vi "Get Test Limits.vi"(10 "Operation Mode":string="Production", 11 "Variant":string="MID") -> (0 "Section6":T1, 1 "Section5":T3, 2 "Section3":T4, 3 "Section2":T5)   [LabVIEW 2025]
uses:
  Controls/Section 2.ctl
  Controls/Limits.ctl
  Controls/Section 3.ctl
  Controls/Section 5.ctl
  Controls/Section 6.ctl
  <vilib>/Utility/file.llb/Read Delimited Spreadsheet (string).vi
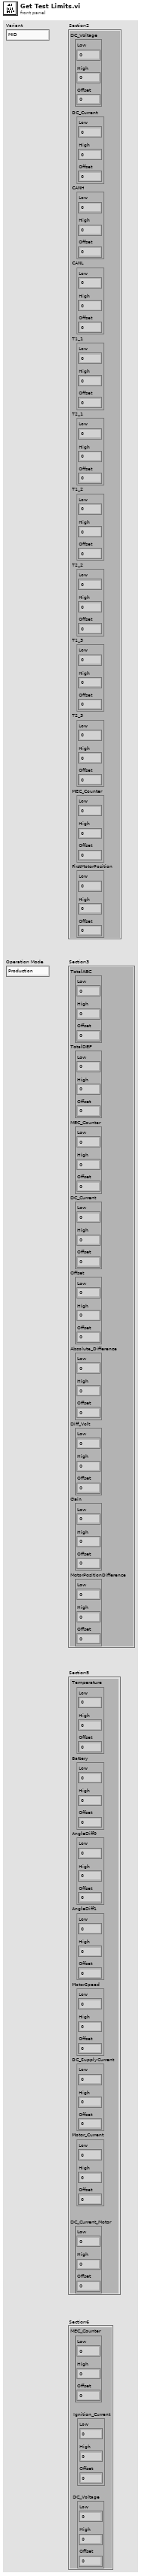
[diagram p1: front panel]
types:
  T1 = typedef "Section 6.ctl" = cluster{"MEC_Counter":T2, "Ignition_Current":T2, "DC_Voltage":T2}
  T2 = typedef "Limits.ctl" = cluster{"Low":dbl, "High":dbl, "Offset":dbl}
  T3 = typedef "Section 5.ctl" = cluster{"Temperature":T2, "Battery":T2, "AngleDiff0":T2, "AngleDiff1":T2, "MotorSpeed":T2, "DC_SupplyCurrent":T2, "Motor_Current":T2, "DC_Current_Motor":T2}
  T4 = typedef "Section 3.ctl" = cluster{"TotalABC":T2, "TotalDEF":T2, "MEC_Counter":T2, "DC_Current":T2, "Offset":T2, "Absolute_Difference":T2, "Diff_Volt":T2, "Gain":T2, "MotorPositionDifference":T2}
  T5 = typedef "Section 2.ctl" = cluster{"DC_Current":T2, "CANH":T2, "CANL":T2, "T1_1":T2, "T2_1":T2, "T1_2":T2, "T2_2":T2, "T1_3":T2, "T2_3":T2, "MEC_Counter":T2, "FirstMotorPosition":T2, "DC_Voltage":T2}
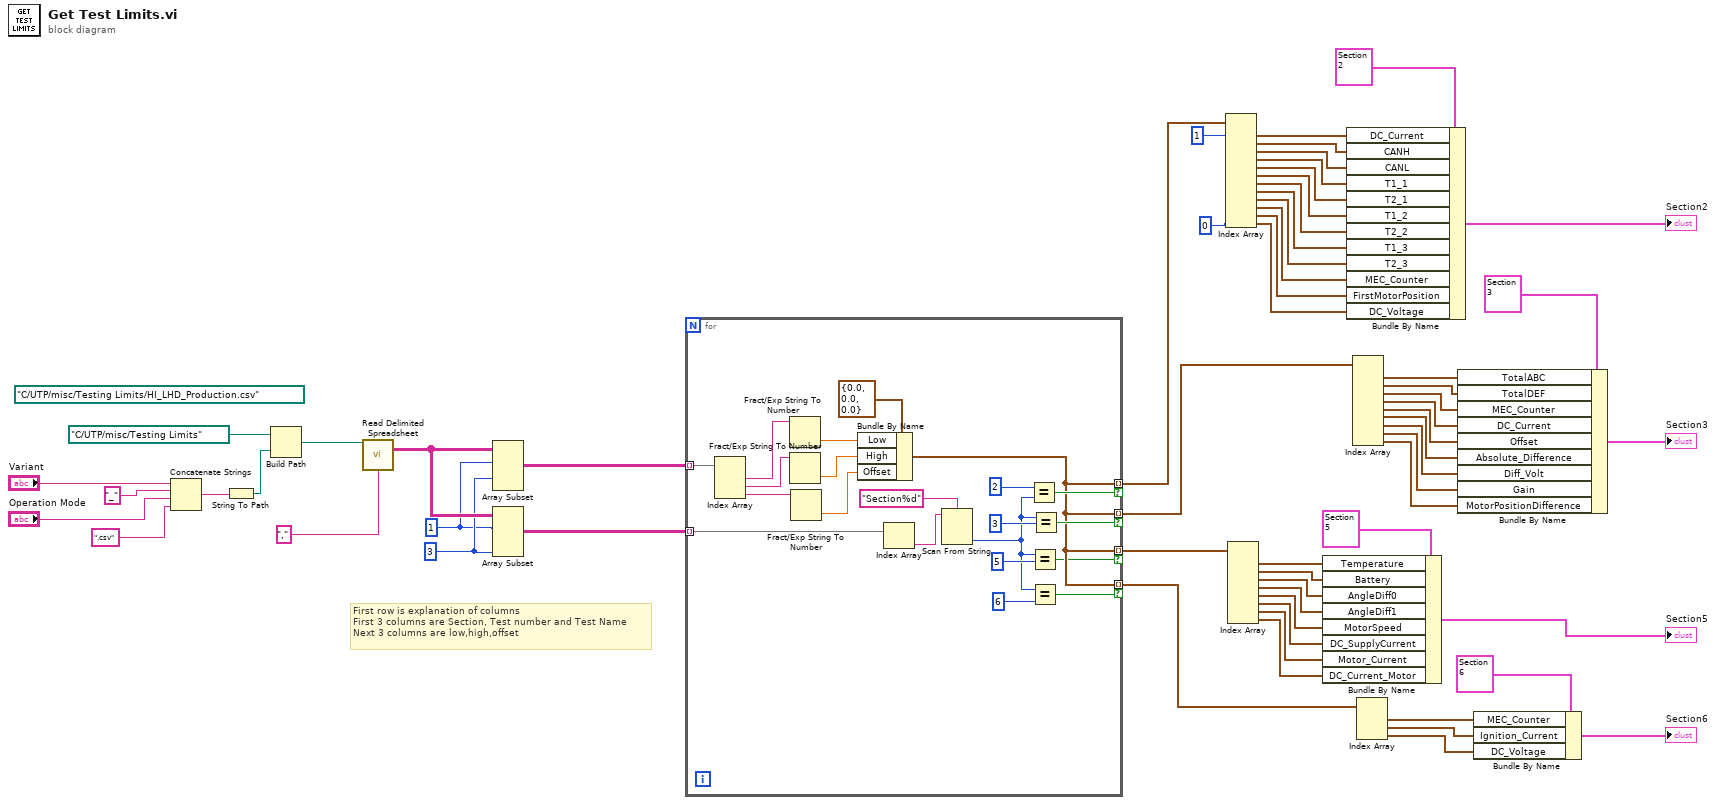
[diagram p0: block diagram]
diagram:
  w57 = 1 ("index")
  w58 = 3 ("index")
  (unwired) path "C:/UTP/misc/Testing Limits/HI_LHD_Production.csv" ("file path (dialog if empty)")
  # "First row is explanation of columns\nFirst 3 columns are Section, Test number and Test Name\nNext 3 columns are low,high,offset"
  n1 = Concatenate Strings("Variant", "_" ("string"), "Operation Mode", ".csv" ("string")) -> (w53:string)
  n2 = String To Path(string=w53) -> (path=w50:path)
  n3 = Build Path(base path=path "C:/UTP/misc/Testing Limits" ("file path (dialog if empty)"), name or relative path=w50) -> (appended path=w49:path)
  n4 = call-poly <vilib>:"Read Delimited Spreadsheet.vi"("file path (dialog if empty)"=w49, "delimiter (\\t)"="," ("delimiter (\\t)")) -> ("all rows"=w59:string[][])  [unwired: 8 in, 5 out]
  n5 = Array Subset(array=w59, index (row)=w57, index (col)=w58) -> (w48:string[][])  [unwired: 2 in]
  n6 = Array Subset(array=w59, index (row)=w57, length (col)=w58) -> (w47:string[][])  [unwired: 2 in]
  n7 = for {
    tunnel: w48 -> [w81] mode=indexing
    tunnel: w47 -> [w77] mode=indexing
    tunnel: [w65] -> w45 mode=indexing if=w69
    tunnel: [w65] -> w32 mode=indexing if=w68
    tunnel: [w65] -> w22 mode=indexing if=w64
    tunnel: [w65] -> w6 mode=indexing if=w61
    n8 = Index Array(array=w81) -> (element #1=w80:string, element #2=w79:string, element #3=w78:string)  [unwired: 3 in]
    n9 = Fract/Exp String To Number(string=w80) -> (number=w72:dbl)  [unwired: 3 in, 1 out]
    n10 = Fract/Exp String To Number(string=w79) -> (number=w71:dbl)  [unwired: 3 in, 1 out]
    n11 = Fract/Exp String To Number(string=w78) -> (number=w70:dbl)  [unwired: 3 in, 1 out]
    n12 = Bundle By Name(cluster=T2 {"Low"=0.0, "High"=0.0, "Offset"=0.0}, "Low"=w72, "High"=w71, "Offset"=w70) -> (w65:T2)
    n13 = Index Array(array=w77) -> (element=w66:string)  [unwired: 1 in]
    n14 = Scan From String(format string="Section%d", input string=w66) -> (output 1=w63:i32)  [unwired: 3 in, 3 out]
    n15 = Equal?(x=2 ("y"), y=w63) -> (x = y?=w69:bool)
    n16 = Equal?(x=w63, y=5) -> (x = y?=w64:bool)
    n17 = Equal?(x=w63, y=6) -> (x = y?=w61:bool)
    n18 = Equal?(x=w63, y=3) -> (x = y?=w68:bool)
  }
  n19 = Index Array(array=w45, index #1=1 ("index"), index #12=0 ("index")) -> (element #1=w44:T2, element #2=w43:T2, element #3=w42:T2, element #4=w41:T2, element #5=w40:T2, element #6=w39:T2, element #7=w38:T2, element #8=w37:T2, element #9=w35:T2, element #10=w36:T2, element #11=w34:T2, element #12=w7:T2)  [unwired: 10 in]
  n20 = Index Array(array=w22) -> (element #1=w20:T2, element #2=w19:T2, element #3=w18:T2, element #4=w17:T2, element #5=w16:T2, element #6=w15:T2, element #7=w14:T2, element #8=w13:T2)  [unwired: 8 in]
  n21 = Bundle By Name(cluster=T3 {"Temperature"={"Low"=0.0, "High"=0.0, "Offset"=0.0}, "Battery"={"Low"=0.0, "High"=0.0, "Offset"=0.0}, "AngleDiff0"={"Low"=0.0, "High"=0.0, "Offset"=0.0}, "AngleDiff1"={"Low"=0.0, "High"=0.0, "Offset"=0.0}, "MotorSpeed"={"Low"=0.0, "High"=0.0, "Offset"=0.0}, "DC_SupplyCurrent"={"Low"=0.0, "High"=0.0, "Offset"=0.0}, "Motor_Current"={"Low"=0.0, "High"=0.0, "Offset"=0.0}, "DC_Current_Motor"={"Low"=0.0, "High"=0.0, "Offset"=0.0}} ("Section5"), "Temperature"=w20, "Battery"=w19, "AngleDiff0"=w18, "AngleDiff1"=w17, "MotorSpeed"=w16, "DC_SupplyCurrent"=w15, "Motor_Current"=w14, "DC_Current_Motor"=w13) -> (→"Section5":T3)
  n22 = Bundle By Name(cluster=T5 {"DC_Current"={"Low"=0.0, "High"=0.0, "Offset"=0.0}, "CANH"={"Low"=0.0, "High"=0.0, "Offset"=0.0}, "CANL"={"Low"=0.0, "High"=0.0, "Offset"=0.0}, "T1_1"={"Low"=0.0, "High"=0.0, "Offset"=0.0}, "T2_1"={"Low"=0.0, "High"=0.0, "Offset"=0.0}, "T1_2"={"Low"=0.0, "High"=0.0, "Offset"=0.0}, "T2_2"={"Low"=0.0, "High"=0.0, "Offset"=0.0}, "T1_3"={"Low"=0.0, "High"=0.0, "Offset"=0.0}, "T2_3"={"Low"=0.0, "High"=0.0, "Offset"=0.0}, "MEC_Counter"={"Low"=0.0, "High"=0.0, "Offset"=0.0}, "FirstMotorPosition"={"Low"=0.0, "High"=0.0, "Offset"=0.0}, "DC_Voltage"={"Low"=0.0, "High"=0.0, "Offset"=0.0}} ("Section2"), "DC_Current"=w44, "CANH"=w43, "CANL"=w42, "T1_1"=w41, "T2_1"=w40, "T1_2"=w39, "T2_2"=w38, "T1_3"=w37, "T2_3"=w35, "MEC_Counter"=w36, "FirstMotorPosition"=w34, "DC_Voltage"=w7) -> (→"Section2":T5)
  n23 = Index Array(array=w32) -> (element #1=w31:T2, element #2=w30:T2, element #3=w29:T2, element #4=w28:T2, element #5=w27:T2, element #6=w26:T2, element #7=w25:T2, element #8=w24:T2, element #9=w23:T2)  [unwired: 9 in]
  n24 = Index Array(array=w6) -> (element #1=w4:T2, element #2=w3:T2, element #3=w2:T2)  [unwired: 3 in]
  n25 = Bundle By Name(cluster=T4 {"TotalABC"={"Low"=0.0, "High"=0.0, "Offset"=0.0}, "TotalDEF"={"Low"=0.0, "High"=0.0, "Offset"=0.0}, "MEC_Counter"={"Low"=0.0, "High"=0.0, "Offset"=0.0}, "DC_Current"={"Low"=0.0, "High"=0.0, "Offset"=0.0}, "Offset"={"Low"=0.0, "High"=0.0, "Offset"=0.0}, "Absolute_Difference"={"Low"=0.0, "High"=0.0, "Offset"=0.0}, "Diff_Volt"={"Low"=0.0, "High"=0.0, "Offset"=0.0}, "Gain"={"Low"=0.0, "High"=0.0, "Offset"=0.0}, "MotorPositionDifference"={"Low"=0.0, "High"=0.0, "Offset"=0.0}} ("Section3"), "TotalABC"=w31, "TotalDEF"=w30, "MEC_Counter"=w29, "DC_Current"=w28, "Offset"=w27, "Absolute_Difference"=w26, "Diff_Volt"=w25, "Gain"=w24, "MotorPositionDifference"=w23) -> (→"Section3":T4)
  n26 = Bundle By Name(cluster=T1 {"MEC_Counter"={"Low"=0.0, "High"=0.0, "Offset"=0.0}, "Ignition_Current"={"Low"=0.0, "High"=0.0, "Offset"=0.0}, "DC_Voltage"={"Low"=0.0, "High"=0.0, "Offset"=0.0}}, "MEC_Counter"=w4, "Ignition_Current"=w3, "DC_Voltage"=w2) -> (→"Section6":T1)
